vi "Control Panel Controller.vi"(8 "error in":errorcluster) -> ()   [LabVIEW 2019]
doc: "This VI executes continuously carrying out the current operation and responding to updates or new operations. It will often contain the timing or control code that is difficult to place directly in TeleOp. This VI generally opens all sensors and motors and isolates the rest of the robot code from knowing how the operations are carried out."
uses:
  <vilib>/Rock Robotics/WPI/Framework/Completion Status.ctl
  Control Panel Setpoints.ctl
  Control Panel Operations.ctl
  <vilib>/Rock Robotics/SystemInterfaces/i2clib/i2c_bus.ctl
  <vilib>/Rock Robotics/Network Tables/NT Write Boolean.vi
panel:
  out "Matched Color Name":string
  out "Match Confidence":dbl
  out "Measured Color":cluster{"R":dbl, "G":dbl, "B":dbl}
  out "error out":errorcluster
  out "Proximity":u16(graph)
  out "Color":u32(colorbox)
  in  "I2C Bus":T1
  in  "Blue Calibration":cluster{"R":dbl, "G":dbl, "B":dbl}={"R"=0.143, "G"=0.427, "B"=0.429}
  in  "Green Calibration":cluster{"R":dbl, "G":dbl, "B":dbl}={"R"=0.197, "G"=0.561, "B"=0.24}
  in  "Red Calibration":cluster{"R":dbl, "G":dbl, "B":dbl}={"R"=0.561, "G"=0.323, "B"=0.114}
  in  "Yellow Calibration":cluster{"R":dbl, "G":dbl, "B":dbl}={"R"=0.361, "G"=0.524, "B"=0.113}
  in  "Interactive Values":T2
  out "Current\nCmd":string
  in  "Buttons":cluster{"Execute Cmd":bool, "Abort Cmd":bool}
  out "Command Timing":cluster{"Start Time (ms)":u32, "Iterations":i32}
  out "Status":T4
  # "Tip: It may be helpful to observe inputs and sensor values.\nYou may also want to display tuning or debugging controls."
  # "Interactive Command: You may fill in the settings for a command\nand schedule it with the Execute button. You can observe and abort\nany command while fine tuning the code for the controller."
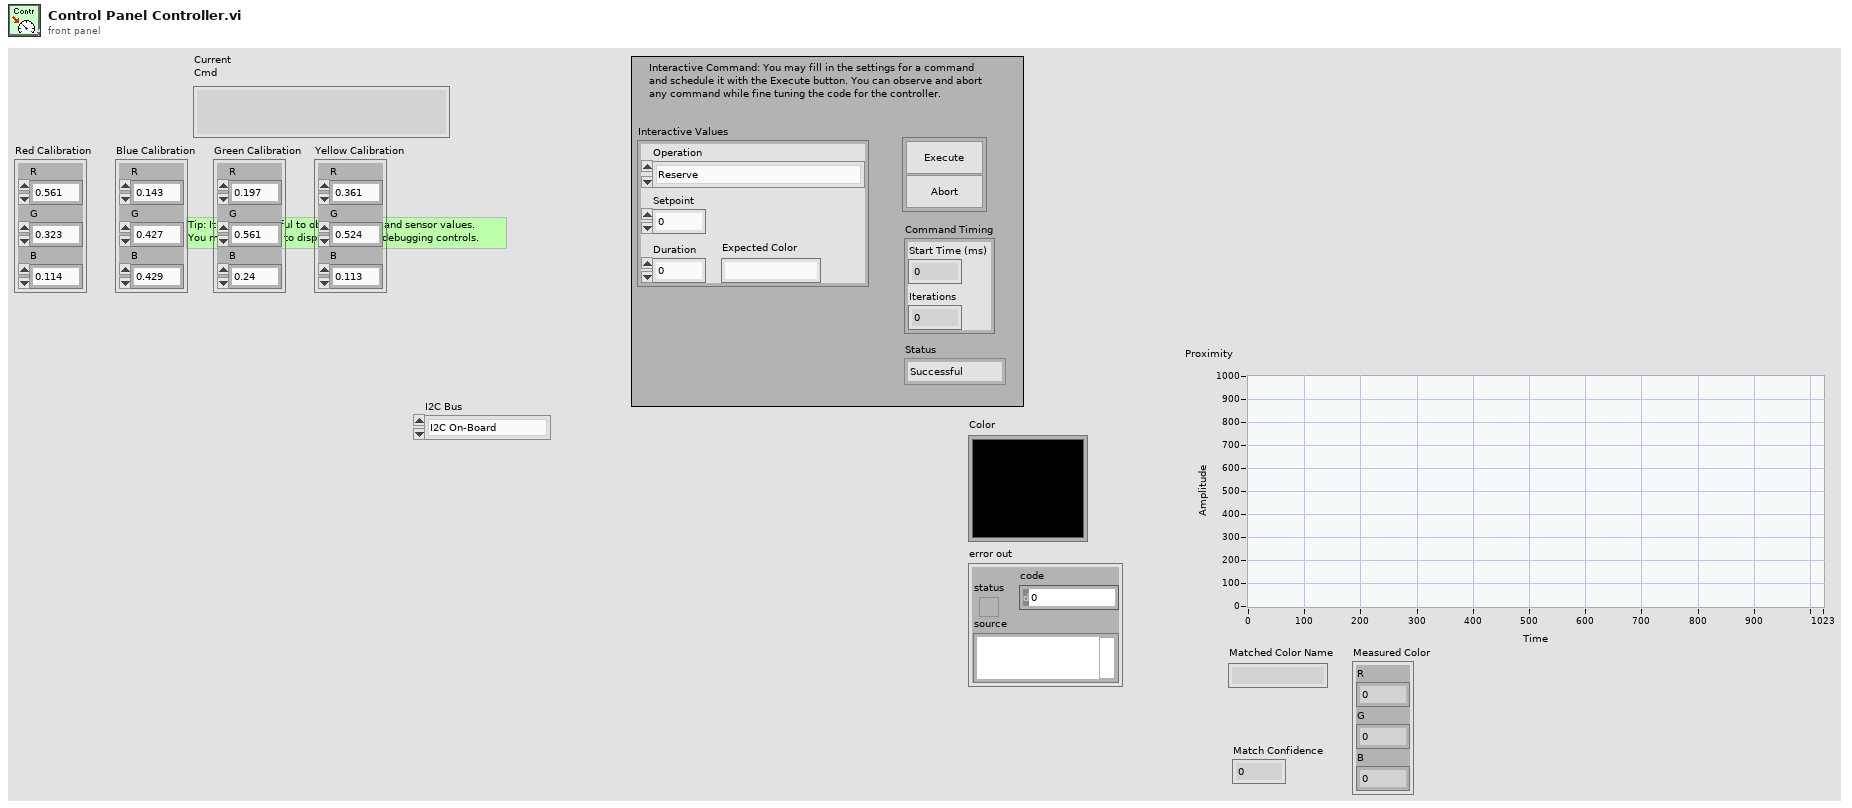
[diagram p1: front panel]
types:
  T1 = typedef "i2c_bus.ctl" = enum16{"I2C On-Board", "I2C MXP", "Invalid"}
  T2 = typedef "Control Panel Setpoints.ctl" = cluster{"Operation":T3, "Setpoint":dbl, "Duration":dbl, "Expected Color":string}
  T3 = typedef "Control Panel Operations.ctl" = enum16{"Reserve", "Read Current", "Immediate", "Rotation control", "Color control"}
  T4 = typedef "Completion Status.ctl" = enum16{"Successful", "Aborted", "Incomplete"}
  T5 = typedef "Color Sensor V3 DevRef.ctl" = cluster{"I2CDevRef":T6}
  T6 = typedef "WPI_I2CDevRef.ctl" = cluster{"DevStatus":errorcluster, "Device Address":u8, "Handle":i32, "I2C Bus":T1}
  T7 = typedef "Command Status Info.ctl" = cluster{"Name":string, "Status":T4, "notifier out":T8}
  T8 = typedef "Completion Notifier.ctl" = refnum<notifier>
  T9 = cluster{"Current Command":T2, "Command Timing":cluster{"Start Time (ms)":u32, "Iterations":i32}, "Command Arguments":cluster{"Command Info":T7, "Description":string, "Default Command":T2, "queue out":refnum<queue>, "Subsystem Name":string}}
  T10 = typedef "WPI_MotorControlDeviceRef.ctl" = cluster{"DeviceStatus":errorcluster, "Type":T11, "PWM":cluster{"PWM Channel":T12, "DeadBand":T13}, "CAN":cluster{"Device Number":u8, "SetOutput VI Ref":variant, "GetOutput VI Ref":variant, "Enable VI Ref":variant, "Disable VI Ref":variant, "Data":variant}, "Invert":bool, "DIO PWM":cluster{"PWM \"Enable\" Channel":T12, "DIOChannel":T14, "PWM Rate":dbl}}
  T11 = typedef "WPI_MotorControlType.ctl" = enum16{"PWM", "CAN", "DIO PWM"}
  T12 = typedef "FPGA_DIOPWMChannel.ctl" = enum8{"PWM 0", "PWM 1", "PWM 2", "PWM 3", "PWM 4", "PWM 5", "PWM 6", "PWM 7", "PWM 8", "PWM 9", "PWM MXP 0", "PWM MXP 1", "PWM MXP 2", "PWM MXP 3", "PWM MXP 4", "PWM MXP 5", "PWM MXP 6", "PWM MXP 7", "PWM MXP 8", "PWM MXP 9", "Invalid"}
  T13 = typedef "WPI_PWMDeadband.ctl" = cluster{"Name":string, "maxPositivePwm":i32, "minPositivePwm":i32, "centerPwm":i32, "maxNegativePwm":i32, "minNegativePwm":i32, "angularRange":u16}
  T14 = typedef "FPGA_DIOChannel.ctl" = enum8{"DIO 0", "DIO 1", "DIO 2", "DIO 3", "DIO 4", "DIO 5", "DIO 6", "DIO 7", "DIO 8", "DIO 9", "DIO MXP 0", "DIO MXP 1", "DIO MXP 2", "DIO MXP 3", "DIO MXP 4", "DIO MXP 5", "DIO MXP 6", "DIO MXP 7", "DIO MXP 8", "DIO MXP 9", "DIO MXP 10", "DIO MXP 11", "DIO MXP 12", "DIO MXP 13", "DIO MXP 14", "DIO MXP 15", "SPI Port CS1", "SPI Port CS2", "SPI Port CS3", "SPI Port MISO", "SPI Port MOSI", "Invalid"}
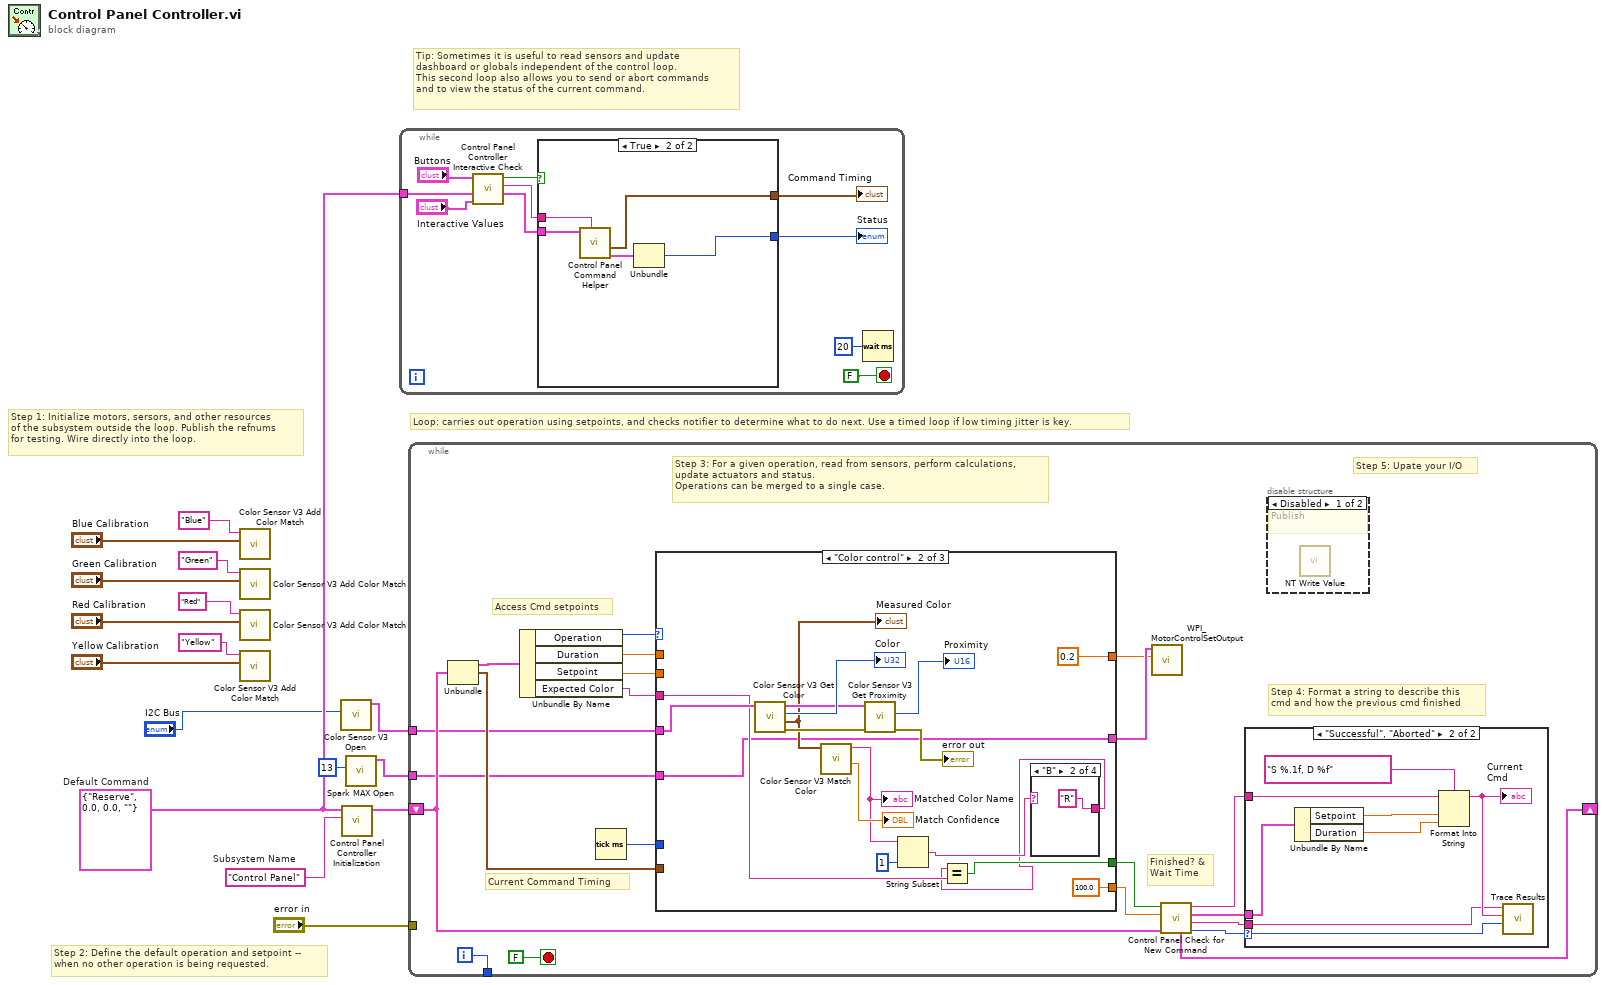
[diagram p0: block diagram]
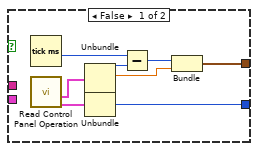
[diagram p2: hidden frame]
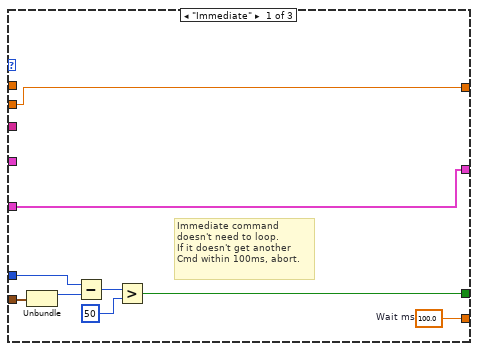
[diagram p5: hidden frame]
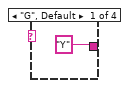
[diagram p6: hidden frame]
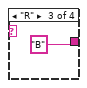
[diagram p7: hidden frame]
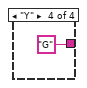
[diagram p8: hidden frame]
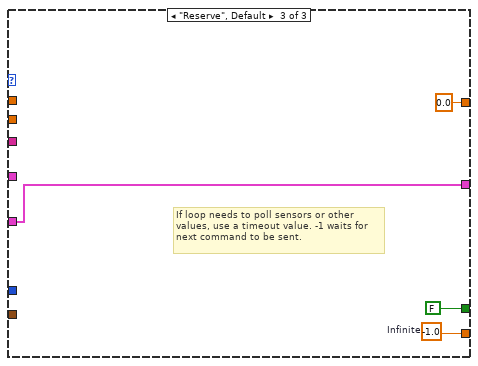
[diagram p9: hidden frame]
diagram:
  w13 = T2 {"Operation"=enum."Reserve", "Setpoint"=0.0, "Duration"=0.0, "Expected Color"=""}  # Default Command
  w14 = "Control Panel"  # Subsystem Name
  # "Tip: Sometimes it is useful to read sensors and update\ndashboard or globals independent of the control loop.\nThis second loop also allows you to send or abort commands\nand to view the status of the current command."
  # "Step 2: Define the default operation and setpoint --\nwhen no other operation is being requested."
  # "Step 1: Initialize motors, sersors, and other resources\nof the subsystem outside the loop. Publish the refnums\nfor testing. Wire directly into the loop."
  # "Loop: carries out operation using setpoints, and checks notifier to determine what to do next. Use a timed loop if low timing jitter is key."
  n1 = call <vilib>:"Color Sensor V3 Add Color Match.vi"("Color"="Blue Calibration", "Name"="Blue") -> ()  [unwired: 10 in]
  n2 = call <vilib>:"Color Sensor V3 Add Color Match.vi"("Color"="Green Calibration", "Name"="Green") -> ()  [unwired: 10 in]
  n3 = call <vilib>:"Color Sensor V3 Add Color Match.vi"("Color"="Red Calibration", "Name"="Red") -> ()  [unwired: 10 in]
  n4 = call <vilib>:"Color Sensor V3 Add Color Match.vi"("Color"="Yellow Calibration", "Name"="Yellow") -> ()  [unwired: 10 in]
  n5 = call <vilib>:"Color Sensor V3 Open.vi"("I2C Bus"="I2C Bus") -> ("ColorSensorDevRef"=w3:T5)  [unwired: 9 in, 1 out]
  n6 = call "Control Panel Controller Initialization.vi"("Subsystem Name"=w14, "Default Command"=w13) -> ("Current Command"=w15:T9)  [unwired: 9 in]
  n7 = call <vilib>:"Spark MAX Open.vi"("Device Number"=u8 13) -> ("MotorControlDeviceRef"=w1:T10)  [unwired: 9 in, 1 out]
  n8 = while {
    tunnel: w13 -> [w23]
    stop <- FALSE stop-if-true
    n9 = call "Control Panel Controller Interactive Check.vi"("Interactive Command in"="Interactive Values", "Default Command"=w23, "Buttons"="Buttons") -> ("Interactive Command out"=w20:T2, "Trace String"=w21:string, "Schedule"=w22:bool)  [unwired: 6 in]
    n10 = case shown="True" w22 {
      tunnel: [w34 w39] -> w19
      tunnel: w20 -> [_ w37]
      tunnel: [w30 w35] -> w18
      tunnel: w21 -> [_ w38]
      frame False {
        n11 = Tick Count (ms)() -> (millisecond timer value=w29:u32)
        n12 = call "Read Control Panel Operation.vi"() -> ("Command Info"=w27:T7, "SubSystem Data"=w28:T2)  [unwired: 9 in, 1 out]
        n13 = Unbundle(w28) -> ("Operation"=w33:T3, "Setpoint"=w31:dbl)  [unwired: 2 out]
        n14 = Unbundle(w27) -> ("Status"=w34:T4)  [unwired: 2 out]
        n15 = Subtract(x=w29, y=w33) -> (x-y=w32:u32)
        n16 = Bundle(w32, "Setpoint"=w31) -> (w30:cluster{u32, "Setpoint":dbl})  [unwired: 1 in]
      }
      frame True {
        n17 = call "Control Panel Command Helper.vi"("Description"=w38, "SubSystem Data"=w37) -> ("Command Info Out"=w36:T7, "Command Timing"=w35:cluster{"Start Time (ms)":u32, "Iterations":i32})  [unwired: 7 in, 1 out]
        n18 = Unbundle(w36) -> ("Status"=w39:T4)  [unwired: 2 out]
      }
    }
    "Status" <- w19
    "Command Timing" <- w18
    n19 = Wait (ms)(milliseconds to wait=u32 20) -> ()  [unwired: 1 out]
  }
  n20 = while {
    shift-right: [w52] -> _
    shift-left: w15 -> [w45]
    tunnel: [w59] -> _
    tunnel: "error in" -> [_]
    tunnel: w3 -> [w43]
    tunnel: w1 -> [w42]
    i -> [w59]
    stop <- FALSE stop-if-true
    # "Step 5: Upate your I/O"
    # "Step 4: Format a string to describe this\ncmd and how the previous cmd finished"
    # "Current Command Timing"
    # "Access Cmd setpoints"
    # "Finished? &\nWait Time"
    # "Step 3: For a given operation, read from sensors, perform calculations,\nupdate actuators and status.\nOperations can be merged to a single case."
    n21 = Unbundle(w45) -> ("Current Command"=w58:T2, "Command Timing"=w54:cluster{"Start Time (ms)":u32, "Iterations":i32})  [unwired: 1 out]
    n22 = Unbundle By Name(w58) -> ("Operation"=w57:T3, "Duration"=w56:dbl, "Setpoint"=w53:dbl, "Expected Color"=w44:string)
    n23 = Tick Count (ms)() -> (millisecond timer value=w55:u32)
    n24 = case shown="\"Color control\"" w57 {
      tunnel: [w77 100.0 ("Infinite") w102] -> w50
      tunnel: [w71 w85 FALSE ("ignore previous (F)")] -> w51
      tunnel: w54 -> [w73 _ _]
      tunnel: w56 -> [_ _ _]
      tunnel: w55 -> [w72 _ _]
      tunnel: w53 -> [w70 _ _]
      tunnel: w44 -> [_ w86 _]
      tunnel: w43 -> [_ w87 _]
      tunnel: w42 -> [w69 w83 w100]
      tunnel: [w69 w83 w100] -> w41
      tunnel: [w70 0.2 0.0] -> w40
      frame "Immediate" {
        w77 = 100.0  # Wait ms
        # "Immediate command\ndoesn't need to loop.\nIf it doesn't get another\nCmd within 100ms, abort."
        n25 = Unbundle(w73) -> ("Start Time (ms)"=w76:u32)  [unwired: 1 out]
        n26 = Subtract(x=w72, y=w76) -> (x-y=w75:u32)
        n27 = Greater?(x=w75, y=u8 50 ("Left Motor")) -> (0:w71:bool)
      }
      frame "Color control" {
        n28 = call <vilib>:"Color Sensor V3 Get Color.vi"("ColorSensorDevRef"=w87) -> ("error out"=w93:errorcluster, "Normalized Color"=w90:cluster{"R":dbl, "G":dbl, "B":dbl}, "Color"=→"Color":u32, "ColorSensorDevRef out"=w92:T5)  [unwired: 7 in]
        "Measured Color" <- w90
        n29 = call <vilib>:"Color Sensor V3 Match Color.vi"("Measured Color"=w90) -> ("Confidence"=→"Match Confidence":dbl, "Matched Color Name"=w81:string)  [unwired: 8 in, 1 out]
        "Matched Color Name" <- w81
        n30 = call <vilib>:"Color Sensor V3 Get Proximity.vi"("error in (no error)"=w93, "ColorSensorDevRef"=w92) -> ("error out"=→"error out":errorcluster, "Proximity"=→"Proximity":u16)  [unwired: 7 in, 1 out]
        n31 = String Subset(string=w81, length (rest)=1 ("length (rest)")) -> (substring=w79:string)  [unwired: 1 in]
        n32 = case shown="\"B\"" w79 {
          tunnel: ["Y" "R" "B" "G"] -> w78
          frame "G", Default {
          }
          frame "B" {
          }
          frame "R" {
          }
          frame "Y" {
          }
        }
        n33 = Equal?(x=w78, y=w86) -> (x = y?=w85:bool)
      }
      frame "Reserve", Default {
        w102 = -1.0  # Infinite
        # "If loop needs to poll sensors or other\nvalues, use a timeout value. -1 waits for\nnext command to be sent."
      }
    }
    n34 = call <vilib>:"WPI_MotorControlSetOutput.vi"("Output"=w40, "MotorControlDevRef"=w41) -> ()  [unwired: 7 in, 3 out]
    n35 = call "Control Panel Check for New Command.vi"("Current Command"=w45, "Wait time (ms)"=w50, "Finished?"=w51) -> ("Completion"=w46:T4, "Subsystem Name"=w47:string, "Current Command"=w48:T2, "Initial Trace String"=w49:string, "NextCommand"=w52:T9)  [unwired: 4 in]
    n36 = case shown="\"Successful\", \"Aborted\"" w46 {
      selector: w46 -> [_ w68]
      tunnel: w49 -> [_ w64]
      tunnel: w48 -> [_ w65]
      tunnel: w47 -> [_ w61]
      frame "Incomplete", Default {
        # "Continuing current command"
      }
      frame "Successful", "Aborted" {
        # "Report and setup for next command"
        n37 = Unbundle By Name(w65) -> ("Setpoint"=w67:dbl, "Duration"=w62:dbl)
        n38 = Format Into String(format string="S %.1f, D %f", initial string=w64, w67, w62) -> (resulting string=w63:string)  [unwired: 1 in, 1 out]
        "Current\nCmd" <- w63
        n39 = call <vilib>:"Trace Results.vi"("Status of previous command"=w68, "Description"=w63, "Subsystem"=w61) -> ()  [unwired: 9 in]
      }
    }
    n40 = disable-structure shown="Disabled" {
      frame Disabled {
        # "Publish"
        n41 = call-poly <vilib>:"NT Write Value.vi"() -> ()  [unwired: 11 in, 1 out]
      }
      frame Enabled {
      }
    }
  }
